vi "Write.vi"(8 "error in (no error)":errorcluster, 10 "Value":T1, 11 "Boolean in":refnum<class "UI-Bus_I8.lvclass">) -> (0 "error out":errorcluster, 3 "Boolean out":refnum<class "UI-Bus_I8.lvclass">)   [LabVIEW 2021, in "UI-Bus_I8.lvclass"]
doc: "Abstract Data Classes 2.1.1.13\nTim Streeter - TSA\nCopyright (c) 2025, TSA"
uses:
  UI-Bus_I8.lvclass
  Type.ctl
  UI-Bus_I8.lvclass/UI-Bus_I8.ctl
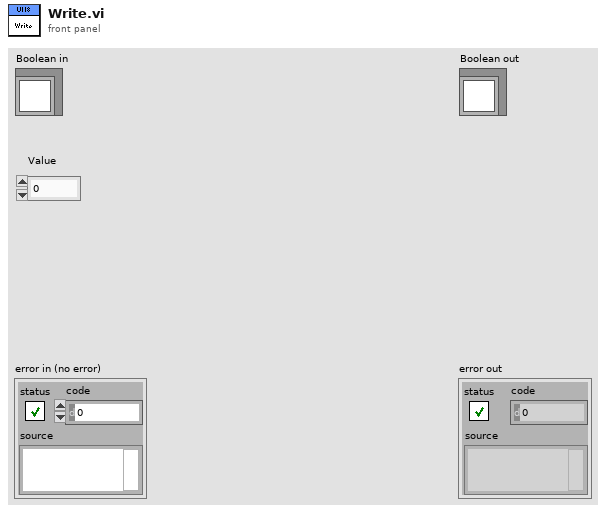
[diagram p1: front panel]
types:
  T1 = typedef "UI-Bus_I8.lvclass/Type.ctl" = i8
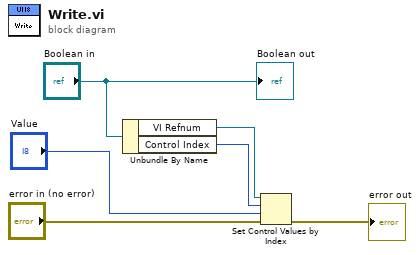
[diagram p0: block diagram]
diagram:
  n1 = Unbundle By Name("Boolean in") -> ("VI Refnum"=w4:refnum<vi>, "Control Index"=w3:i32)
  n2 = Set Control Values by Index(0:w4, 1:w3, 2:"Value", 3:"error in (no error)") -> (11:→"error out":errorcluster)
  "Boolean out" <- "Boolean in"
